vi "rs3_2D Plane fit_sub.vi"(6 "algorithm":T1 items=["SVD", "Givens", "Givens2", "Householder", "LU Decomposition", "Cholesky", "SVD for Rank Deficient H"], 7 "method":T2 items=["Least Square", "Least Absolute Residual", "Bisquare"], 9 "Z":dbl[](array[numeric])=[5.0, 5.1, 5.1, 5.1, 4.9, 5.1, 5.1, 5.0, 5.0], 10 "Y":dbl[](array[numeric])=[0.0, 0.0, 0.0, 1.0, 1.0, 1.0, 2.0, 2.0, 3.0], 11 "X":dbl[](array[numeric])=[1.0, 2.0, 3.0, 1.0, 2.0, 3.0, 1.0, 2.0, 3.0]) -> (0 "Coefficients":dbl[](array[numeric])=[5.057324840764333, 0.002760084925691242, -0.016560509554140346], 1 "mean Z Value":dbl=5.04447078879859 format="%0.2f", 2 "rms error value":dbl=0.06652497327232935 format="%0.4f", 3 "rms %":dbl=1.3187701159862044 format="%0.4f", 4 "Deviation":dbl[](array[numeric])=[-0.060084925690023994, 0.037154989384283965, 0.03439490445859228, 0.05647558386411511, -0.14628450106157498, 0.05095541401273351, 0.07303609341825634, -0.029723991507434988, -0.01592356687898544], 5 "Best Fit":dbl[](array[numeric])=[5.060084925690024, 5.062845010615716, 5.065605095541407, 5.0435244161358845, 5.046284501061575, 5.049044585987266, 5.026963906581743, 5.029723991507435, 5.015923566878985])   [LabVIEW 2017, in "libRealSense3.lvlib"]
uses:
  <vilib>/Analysis/6fits.llb/Curve Fitting Criteria.ctl
  <vilib>/Analysis/6fits.llb/General Linear Fit Algorithm.ctl
  <vilib>/Analysis/5stat.llb/RMS (DBL).vi
  <vilib>/Analysis/baseanly.llb/Mean (DBL).vi
  libRealSense3.lvlib
  <vilib>/Analysis/NI_AALPro.lvlib
  <vilib>/Analysis/NI_AALBase.lvlib
panel:
  # "INPUT DATA"
  # "PLANE FIT"
  # "Z= A +B*x+C*y"
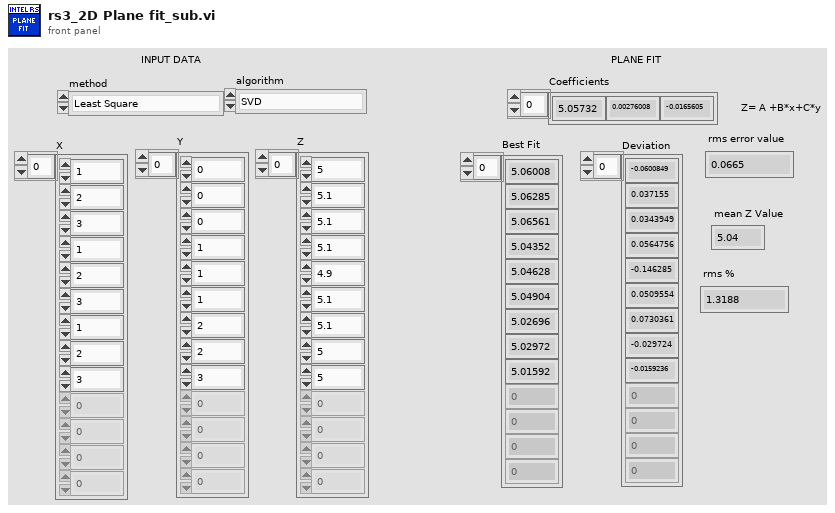
[diagram p1: front panel]
types:
  T1 = typedef "NI_AALPro.lvlib/General Linear Fit Algorithm.ctl" = u16
  T2 = typedef "NI_AALPro.lvlib/Curve Fitting Criteria.ctl" = u16
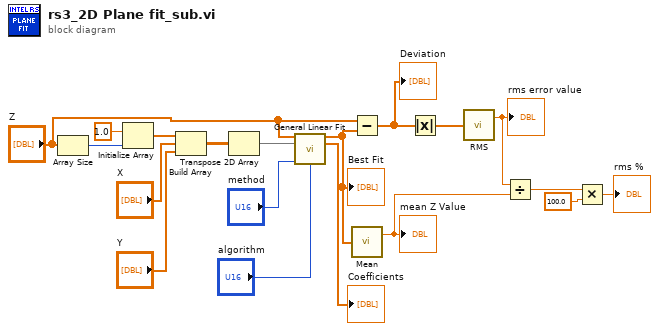
[diagram p0: block diagram]
diagram:
  n1 = Array Size(array="Z") -> (size(s)=w19:i32)
  n2 = Initialize Array(1.0 ("element"), w19) -> (w17:dbl[])
  n3 = Build Array(w17, "X", "Y") -> (w4:dbl[][])
  n4 = Transpose 2D Array(2D array=w4) -> (transposed array=w16:dbl[][])
  n5 = call <vilib>:"General Linear Fit.vi"("Y"="Z", "H"=w16, "method"="method", "algorithm"="algorithm") -> ("Best Fit"=w10:dbl[], "Coefficients"=→"Coefficients":dbl[])  [unwired: 6 in, 4 out]
  "Best Fit" <- w10
  n6 = Subtract(x="Z", y=w10) -> (x-y=w12:dbl[])
  "Deviation" <- w12
  n7 = call-poly <vilib>:"Mean.vi"("X"=w10) -> ("mean"=w8:dbl)  [unwired: 1 out]
  "mean Z Value" <- w8
  n8 = Absolute Value(x=w12) -> (abs(x)=w11:dbl[])
  n9 = call-poly <vilib>:"RMS.vi"("X"=w11) -> ("rms value"=w9:dbl)  [unwired: 1 out]
  "rms error value" <- w9
  n10 = Divide(x=w9, y=w8) -> (x/y=w7:dbl)
  n11 = Multiply(x=w7, y=100.0) -> (x*y=→"rms %":dbl)
